vi "Mavg method_v2.vi"(4 "Encoder Position":i16, 6 "D_d_pre":fxp<+/-,49,33>, 7 "Tick Count (usec)":i16, 8 "Encoder Position array_pre":i32[](array[numeric])=[0, 0, 0, 0, 0, 0, 0, 0, 0, 0, 0, 0, 0, 0, 0, 0, 0, 0, 0, 0, 0, 0, 0, 0, 0], 9 "Tc array_pre":i32[](array[numeric])=[0, 0, 0, 0, 0, 0, 0, 0, 0, 0, 0, 0, 0, 0, 0, 0, 0, 0, 0, 0, 0, 0, 0, 0, 0], 10 "Tc_Mavg (usec)":i32) -> (0 "D_d":fxp<+/-,49,33>, 1 "Encoder Position array":i32[](array[numeric]), 2 "Tc array":i32[](array[numeric]), 3 "omega":fxp<+/-,64,35>)   [LabVIEW 2014]
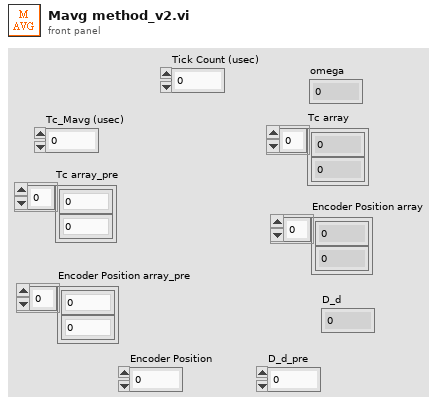
[diagram p1: front panel]
types:
  T1 = cluster{"Encoder Position array_pre[0]":i32, "Encoder Position array_pre[1]":i32, "Encoder Position array_pre[2]":i32, "Encoder Position array_pre[3]":i32, "Encoder Position array_pre[4]":i32, "Encoder Position array_pre[5]":i32, "Encoder Position array_pre[6]":i32, "Encoder Position array_pre[7]":i32, "Encoder Position array_pre[8]":i32, "Encoder Position array_pre[9]":i32, "Encoder Position array_pre[10]":i32, "Encoder Position array_pre[11]":i32, "Encoder Position array_pre[12]":i32, "Encoder Position array_pre[13]":i32, "Encoder Position array_pre[14]":i32, "Encoder Position array_pre[15]":i32, "Encoder Position array_pre[16]":i32, "Encoder Position array_pre[17]":i32, "Encoder Position array_pre[18]":i32, "Encoder Position array_pre[19]":i32, "Encoder Position array_pre[20]":i32, "Encoder Position array_pre[21]":i32, "Encoder Position array_pre[22]":i32, "Encoder Position array_pre[23]":i32, "Encoder Position array_pre[24]":i32}
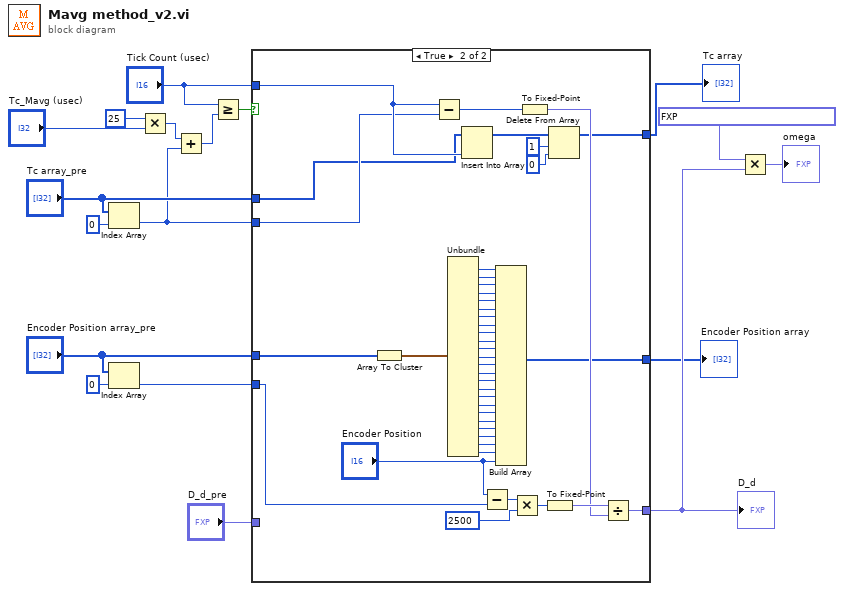
[diagram p0: block diagram]
diagram:
  n1 = Index Array(array="Tc array_pre", index=0) -> (element=w3:i32)
  n2 = Index Array(array="Encoder Position array_pre", index=0) -> (element=w4:i32)
  n3 = Multiply(x=25, y="Tc_Mavg (usec)") -> (x*y=w12:i32)
  n4 = Add(x=w12, y=w3) -> (x+y=w9:i32)
  n5 = Greater Or Equal?(x="Tick Count (usec)", y=w9) -> (x >= y?=w11:bool)
  n6 = case shown="True" w11 {
    tunnel: "Tick Count (usec)" -> [_ w60]
    tunnel: w3 -> [_ w59]
    tunnel: w4 -> [_ w52]
    tunnel: "Tc array_pre" -> [w21 w58]
    tunnel: "Encoder Position array_pre" -> [w20 w24]
    tunnel: [w19 w51] -> w16
    tunnel: [w20 w22] -> w2
    tunnel: [w21 w50] -> w1
    tunnel: "D_d_pre" -> [w19 _]
    frame False {
    }
    frame True {
      n7 = Array To Cluster(array=w24) -> (cluster=w25:T1)
      n8 = Subtract(x=w60, y=w59) -> (x-y=w61:i32)
      n9 = Unbundle(w25) -> ("Encoder Position array_pre[1]"=w26:i32, "Encoder Position array_pre[2]"=w27:i32, "Encoder Position array_pre[3]"=w28:i32, "Encoder Position array_pre[4]"=w29:i32, "Encoder Position array_pre[5]"=w30:i32, "Encoder Position array_pre[6]"=w31:i32, "Encoder Position array_pre[7]"=w32:i32, "Encoder Position array_pre[8]"=w33:i32, "Encoder Position array_pre[9]"=w34:i32, "Encoder Position array_pre[10]"=w35:i32, "Encoder Position array_pre[11]"=w36:i32, "Encoder Position array_pre[12]"=w37:i32, "Encoder Position array_pre[13]"=w38:i32, "Encoder Position array_pre[14]"=w39:i32, "Encoder Position array_pre[15]"=w40:i32, "Encoder Position array_pre[16]"=w41:i32, "Encoder Position array_pre[17]"=w42:i32, "Encoder Position array_pre[18]"=w43:i32, "Encoder Position array_pre[19]"=w44:i32, "Encoder Position array_pre[20]"=w45:i32, "Encoder Position array_pre[21]"=w46:i32, "Encoder Position array_pre[22]"=w47:i32, "Encoder Position array_pre[23]"=w48:i32, "Encoder Position array_pre[24]"=w49:i32)  [unwired: 1 out]
      n10 = Insert Into Array(array=w58, new element=w60) -> (w63:i32[])  [unwired: 1 in]
      n11 = Subtract(x="Encoder Position", y=w52) -> (x-y=w57:i32)
      n12 = Build Array(w26, w27, w28, w29, w30, w31, w32, w33, w34, w35, w36, w37, w38, w39, w40, w41, w42, w43, w44, w45, w46, w47, w48, w49, "Encoder Position") -> (w22:i32[])
      n13 = Multiply(x=w57, y=2500) -> (x*y=w55:i32)
      n14 = To Fixed-Point(number=w61) -> (fixed-point=w53:fxp<+/-,32,32>)  [unwired: 1 in]
      n15 = To Fixed-Point(number=w55) -> (fixed-point=w54:fxp<+/-,32,32>)  [unwired: 1 in]
      n16 = Delete From Array(array=w63, length=1, index=0) -> (array with subset deleted=w50:i32[])  [unwired: 1 out]
      n17 = Divide(x=w54, y=w53) -> (x/y=w51:fxp<+/-,64,33>)
    }
  }
  "D_d" <- w16
  "Tc array" <- w1
  "Encoder Position array" <- w2
  n18 = Multiply(x=fxp<+/-,27,3> 3.1415926218032837, y=w16) -> (x*y=→"omega":fxp<+/-,64,36>)
